vi "Data Handling R2.vi"(0 "Cluster":T1, 11 "Data Buffer":u8[](array[numeric])) -> (1 "Psi (image)":dbl, 2 "Theta (image)":dbl, 3 "Psi array out":i16, 4 "Theta array out":i16, 10 "Time":dbl, 12 "Cx":dbl, 13 "Cy":dbl, 14 "Target array":dbl[][](array[numeric]), 15 "output cluster":T2)   [LabVIEW 2015]
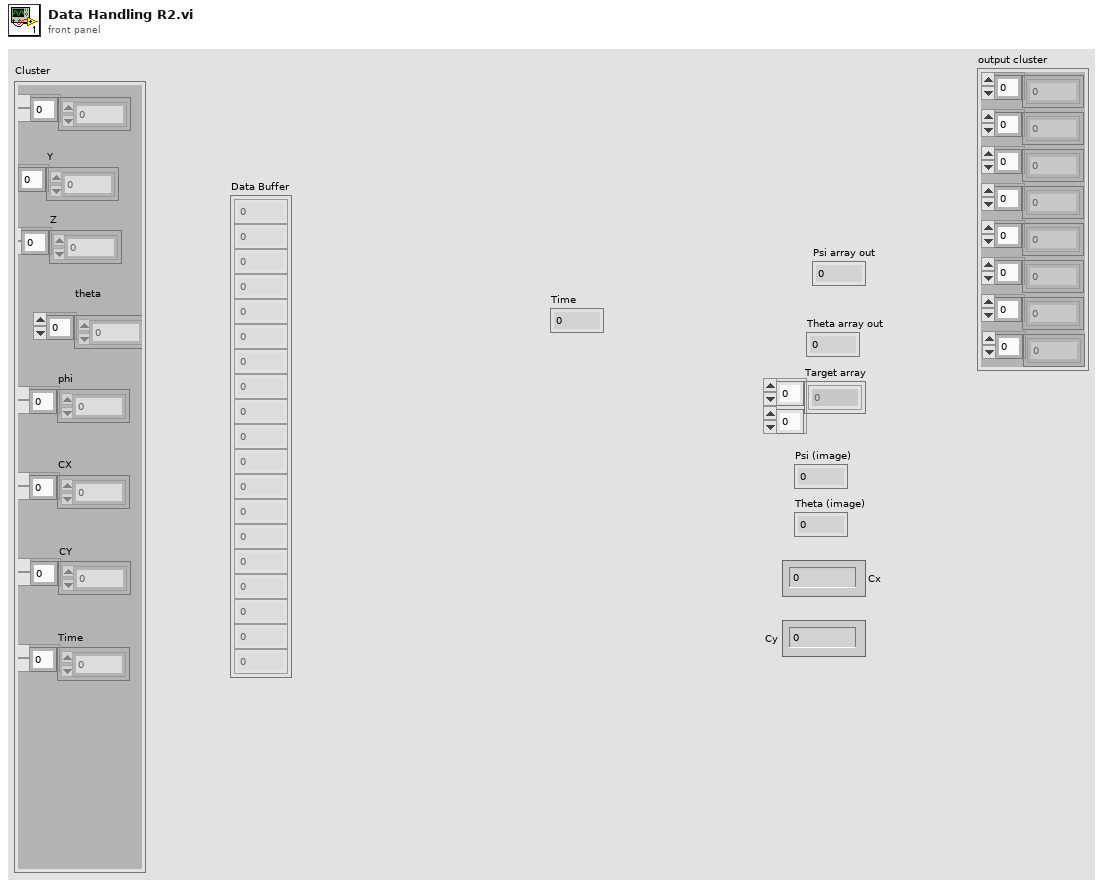
[diagram p1: front panel]
types:
  T1 = cluster{"X":dbl[], "Y":dbl[], "Z":dbl[], "theta":u16[], "phi":u16[], "CX":u16[], "CY":u16[], "Time":dbl[]}
  T2 = cluster{dbl[], dbl[], dbl[], u16[], u16[], u16[], u16[], dbl[]}
  T3 = cluster{"Data Buffer[0]":u8, "Data Buffer[1]":u8, "Data Buffer[2]":u8, "Data Buffer[3]":u8, "Data Buffer[4]":u8, "Data Buffer[5]":u8, "Data Buffer[6]":u8, "Data Buffer[7]":u8, "Data Buffer[8]":u8, "Data Buffer[9]":u8, "Data Buffer[10]":u8, "Data Buffer[11]":u8, "Data Buffer[12]":u8, "Data Buffer[13]":u8, "Data Buffer[14]":u8, "Data Buffer[15]":u8, "Data Buffer[16]":u8}
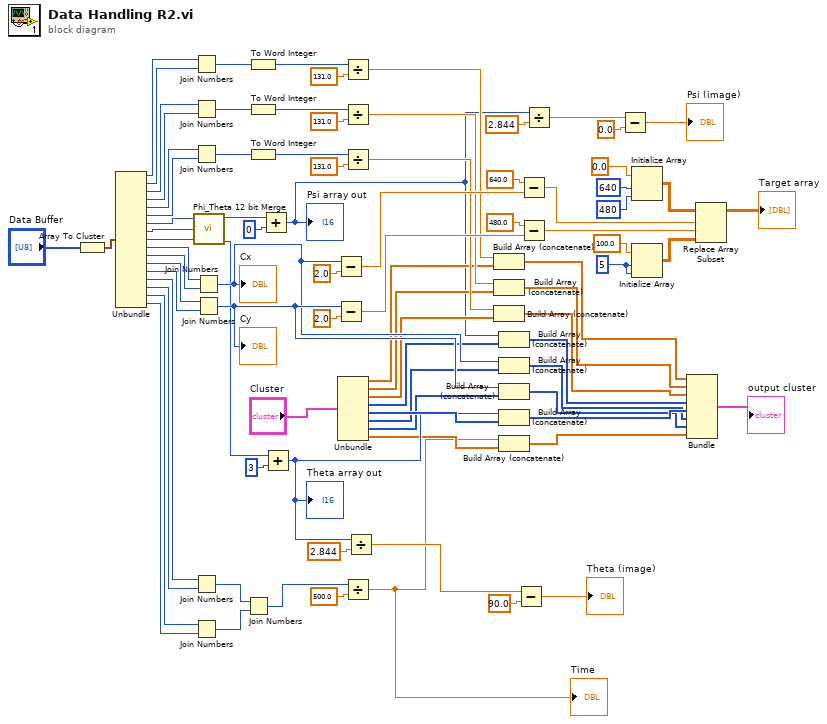
[diagram p0: block diagram]
diagram:
  w65 = 5 ("dimension size")
  n1 = Array To Cluster(array="Data Buffer") -> (cluster=w86:T3)
  n2 = Unbundle(w86) -> ("Data Buffer[0]"=w85:u8, "Data Buffer[1]"=w84:u8, "Data Buffer[2]"=w83:u8, "Data Buffer[3]"=w82:u8, "Data Buffer[4]"=w81:u8, "Data Buffer[5]"=w80:u8, "Data Buffer[6]"=w53:u8, "Data Buffer[7]"=w52:u8, "Data Buffer[8]"=w51:u8, "Data Buffer[9]"=w56:u8, "Data Buffer[10]"=w57:u8, "Data Buffer[11]"=w58:u8, "Data Buffer[12]"=w59:u8, "Data Buffer[13]"=w15:u8, "Data Buffer[14]"=w16:u8, "Data Buffer[15]"=w17:u8, "Data Buffer[16]"=w18:u8)
  n3 = Join Numbers(hi=w85, lo=w84) -> ((hi.lo)=w79:u16)
  n4 = Join Numbers(hi=w83, lo=w82) -> ((hi.lo)=w74:u16)
  n5 = Join Numbers(hi=w81, lo=w80) -> ((hi.lo)=w73:u16)
  n6 = Join Numbers(hi=w15, lo=w16) -> ((hi.lo)=w4:u16)
  n7 = Join Numbers(hi=w17, lo=w18) -> ((hi.lo)=w3:u16)
  n8 = call "Phi_Theta 12 bit Merge.vi"("Phi H/Theta H"=w51, "Theta L"=w52, "Phi L"=w53) -> ("Theta"=w12:u16, "Phi"=w10:u16)  [unwired: 4 in]
  n9 = Join Numbers(hi=w56, lo=w57) -> ((hi.lo)=w60:u16)
  "Cx" <- w60
  n10 = Join Numbers(hi=w58, lo=w59) -> ((hi.lo)=w61:u16)
  "Cy" <- w61
  n11 = Join Numbers(hi=w4, lo=w3) -> ((hi.lo)=w2:u32)
  n12 = To Word Integer(number=w79) -> (16bit integer=w77:i16)
  n13 = To Word Integer(number=w74) -> (16bit integer=w75:i16)
  n14 = To Word Integer(number=w73) -> (16bit integer=w71:i16)
  n15 = Add(x=w10, y=u16 0) -> (x+y=w9:u16)
  "Psi array out" <- w9
  n16 = Add(x=w12, y=u16 3) -> (x+y=w13:u16)
  "Theta array out" <- w13
  n17 = Subtract(x=w60, y=2.0) -> (x-y=w49:dbl)
  n18 = Subtract(x=w61, y=2.0) -> (x-y=w46:dbl)
  n19 = Unbundle("Cluster") -> ("X"=w33:dbl[], "Y"=w32:dbl[], "Z"=w31:dbl[], "theta"=w30:u16[], "phi"=w29:u16[], "CX"=w28:u16[], "CY"=w27:u16[], "Time"=w7:dbl[])
  n20 = Divide(x=w77, y=131.0) -> (x/y=w44:dbl)
  n21 = Divide(x=w75, y=131.0) -> (x/y=w43:dbl)
  n22 = Divide(x=w71, y=131.0) -> (x/y=w42:dbl)
  n23 = Divide(x=w2, y=500.0) -> (x/y=w1:dbl)
  "Time" <- w1
  n24 = Divide(x=w13, y=2.844) -> (x/y=w20:dbl)
  n25 = Build Array (concatenate)(w44, w33) -> (w41:dbl[])
  n26 = Build Array (concatenate)(w43, w32) -> (w40:dbl[])
  n27 = Build Array (concatenate)(w42, w31) -> (w39:dbl[])
  n28 = Build Array (concatenate)(w9, w30) -> (w38:u16[])
  n29 = Build Array (concatenate)(w60, w28) -> (w36:u16[])
  n30 = Build Array (concatenate)(w61, w27) -> (w35:u16[])
  n31 = Build Array (concatenate)(w13, w29) -> (w37:u16[])
  n32 = Build Array (concatenate)(w1, w7) -> (w6:dbl[])
  n33 = Subtract(x=w20, y=90.0) -> (x-y=→"Theta (image)":dbl)
  n34 = Subtract(x=640.0, y=w49) -> (x-y=w48:dbl)
  n35 = Subtract(x=480.0, y=w46) -> (x-y=w45:dbl)
  n36 = Divide(x=w9, y=2.844) -> (x/y=w23:dbl)
  n37 = Subtract(x=w23, y=0.0) -> (x-y=→"Psi (image)":dbl)
  n38 = Initialize Array(0.0 ("element"), 640 ("dimension size"), 480 ("dimension size")) -> (w67:dbl[][])
  n39 = Initialize Array(100.0 ("element"), w65, w65) -> (w64:dbl[][])
  n40 = Bundle(w41, w40, w39, w38, w37, w36, w35, w6) -> (→"output cluster":T2)  [unwired: 1 in]
  n41 = Replace Array Subset(array=w67, new element=w64, index (row)=w48, index (col)=w45) -> (→"Target array":dbl[][])
